vi "Refresh Menus 2013.vi"(8 "error in (no error)":errorcluster) -> (0 "error out":errorcluster)   [LabVIEW 2013]
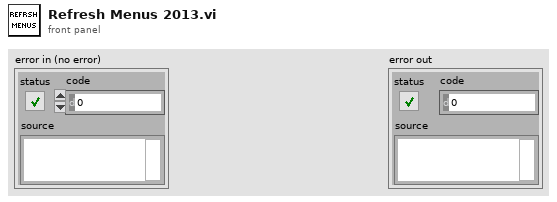
[diagram p1: front panel]
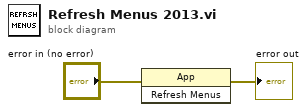
[diagram p0: block diagram]
diagram:
  n1 = invoke class="App" method="Refresh Menus"(error in="error in (no error)") -> (error out=→"error out":errorcluster)  [unwired: 2 in, 2 out]
